vi "Get Channel Index by Name.vi"(8 "error in (no error)":errorcluster, 10 "Channel Name":string, 11 "CIFChannelMng in":refnum<class "CIFChannelMng.lvclass">) -> (0 "error out":errorcluster, 2 "Channel Index":i32=65535, 3 "CIFChannelMng out":refnum<class "CIFChannelMng.lvclass">)   [LabVIEW 2021, in "CIFChannelMng.lvclass"]
uses:
  CIFChannelMng.lvclass
  CIFChannelMng.lvclass/CIFChannelMng.ctl
  CIFUtilities/CIFClocks/Typedef/Errors.ctl
  CIFCore/Common/Utilities/Append Error Location.vi
  CIFCore/Common/CIFCoreCommon.lvlib
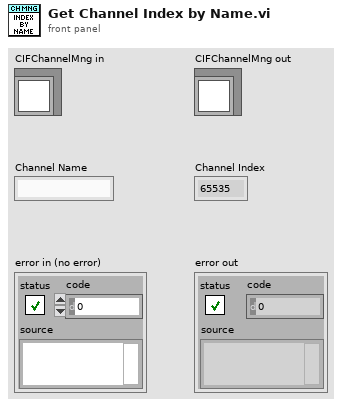
[diagram p1: front panel]
types:
  T1 = typedef "CIFCoreCommon.lvlib/Errors.ctl" = enum16{"Invalid Clock ID", "Long Sleep", "gRPC Server Not Found", "Config Parse", "Timestamp Wrap", "Delayed Execution", "Duplicate Channel", "Missing Channel", "Incorrect Type", "Flatten Error"}
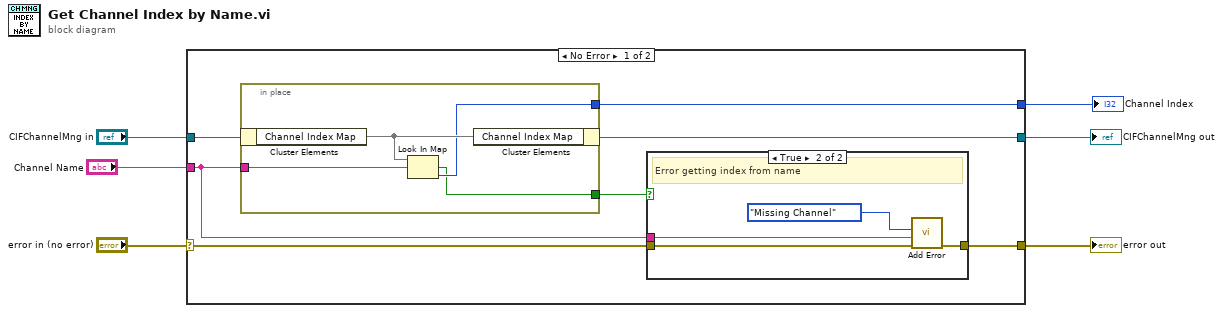
[diagram p0: block diagram]
diagram:
  n1 = case shown="No Error" "error in (no error)" {
    selector: "error in (no error)" -> [w11 w24]
    tunnel: [w10 w24] -> w5
    tunnel: [w9 w23] -> w3
    tunnel: "CIFChannelMng in" -> [w8 w23]
    tunnel: "Channel Name" -> [w13 _]
    tunnel: [w12 _] -> w1
    frame No Error {
      n2 = in-place {
        in-place-border: w13 -> [w14]
        in-place-border: [w16] -> w12
        in-place-border: [w15] -> w7
        n3 = in-place-cluster #1(w8) -> ("Channel Index Map"=w17:map{string, i32})
        n4 = Look In Map(map=w17, key=w14) -> (key not found?=w15:bool, value=w16:i32)  [unwired: 1 in]
        n5 = in-place-cluster #1("Channel Index Map"=w17) -> (w9:refnum<class "CIFChannelMng.lvclass">)
      }
      n6 = case shown="True" w7 {
        tunnel: w11 -> [w18 w22]
        tunnel: [w18 w21] -> w10
        tunnel: w13 -> [_ w19]
        frame False {
          # "no error"
        }
        frame True {
          # "Error getting index from name"
          n7 = call "Add Error.vi"("error in (no error)"=w22, "String to Append"=w19, "Error"=Errors."Missing Channel") -> ("error out"=w21:errorcluster)  [unwired: 8 in]
        }
      }
    }
    frame Error {
    }
  }
  "error out" <- w5
  "CIFChannelMng out" <- w3
  "Channel Index" <- w1
